vi "getImageinfo.vi"(8 "error in (no error)":errorcluster, 11 "params":refnum<class "JSON Value.lvclass">) -> (0 "error out":errorcluster, 3 "data":refnum<class "JSON Value.lvclass">)   [LabVIEW 2017]
uses:
  <vilib>/NI/JSON Support for LabVIEW/JSON Value/JSON Value.lvclass
  ax5.lvclass
  <vilib>/NI/JSON Support for LabVIEW/JSON Value/Object/Get Value/Get Value (String).vi
  <vilib>/NI/JSON Support for LabVIEW/JSON Value/Object/Get Value/Get Value (Numeric).vi
  <vilib>/NI/JSON Support for LabVIEW/JSON Value/New JSON Value/New JSON (Numeric).vi
  <vilib>/NI/JSON Support for LabVIEW/JSON Value/New JSON Value/New JSON (Numeric[]).vi
  <vilib>/NI/JSON Support for LabVIEW/JSON Value/New JSON Value/New JSON ({Value[]}).vi
  <vilib>/NI/NI JSONRPC Server Framework/Classes/Server/JSONRPC Server.lvclass
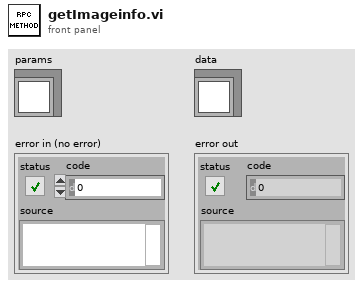
[diagram p1: front panel]
types:
  T1 = typedef "Image Type" = u32
  T2 = cluster{"histogram":u32[], "Minimal Value":sgl, "Maximal Value":sgl, "Starting Value":sgl, "Interval Width":sgl, "Mean Value":sgl, "Standard  Variation":sgl, "Area (pixels)":i32}
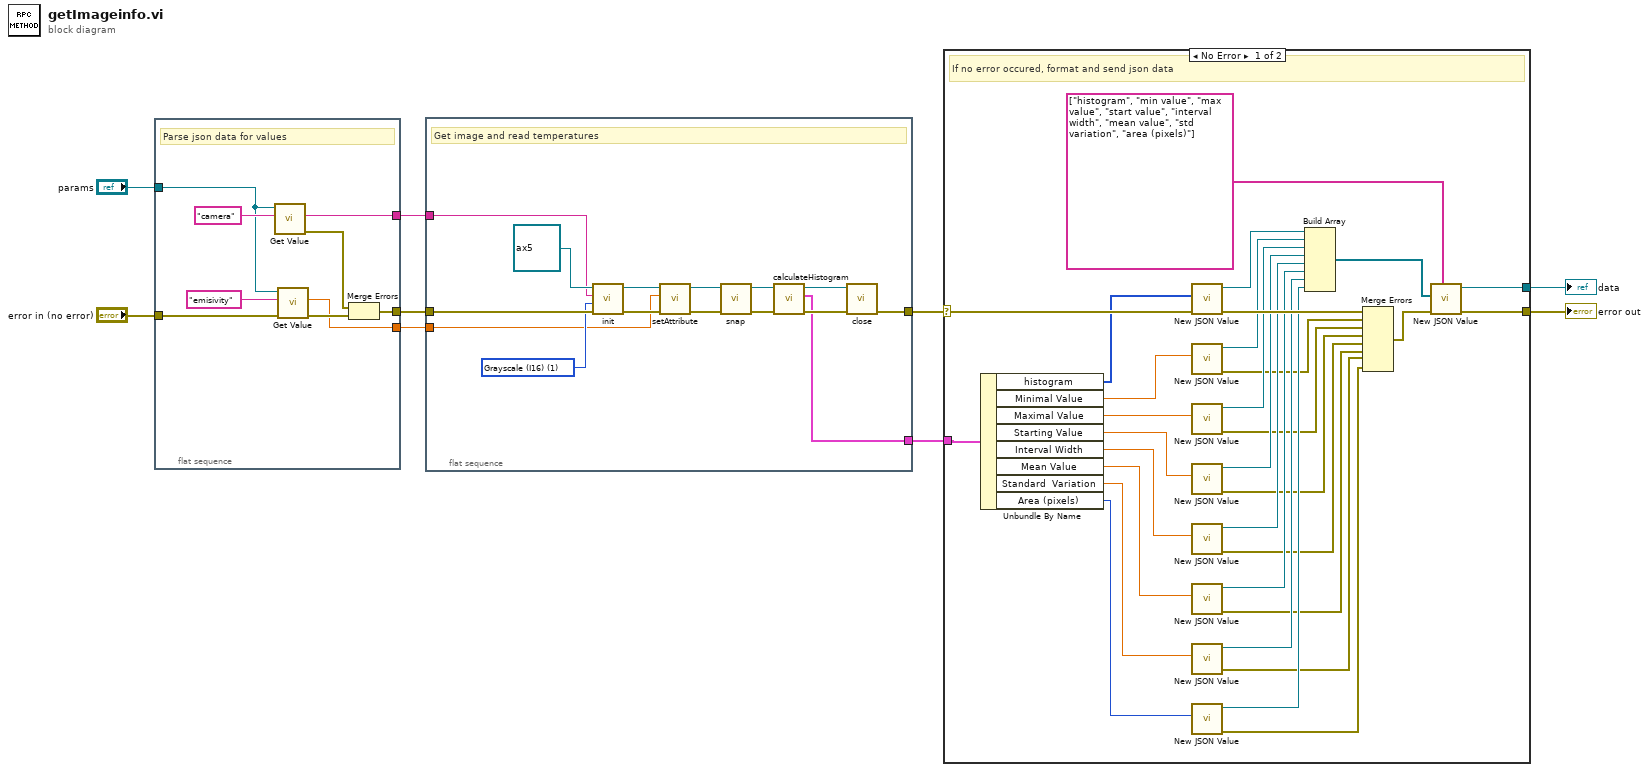
[diagram p0: block diagram]
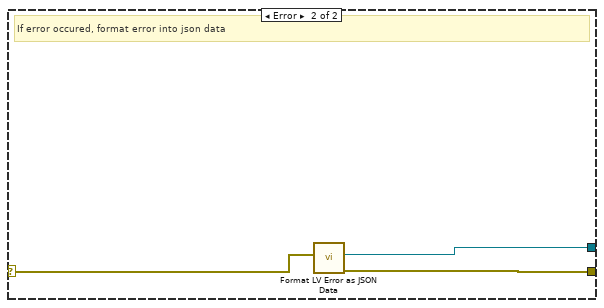
[diagram p2: hidden frame]
diagram:
  n1 = flat-sequence {
    tunnel: "params" -> [w16]
    tunnel: "error in (no error)" -> [w15]
    tunnel: [w12] -> w7
    tunnel: [w11] -> w6
    tunnel: [w10] -> w5
    frame #0 {
      # "Parse json data for values"
      n2 = call-poly <vilib>:"Get Value.vi"("key"="camera", "JSON Value in"=w16) -> ("error out"=w13:errorcluster, "value"=w11:string)  [unwired: 8 in]
      n3 = call-poly <vilib>:"Get Value.vi"("error in (no error)"=w15, "key"="emisivity", "JSON Value in"=w16) -> ("error out"=w14:errorcluster, "value"=w10:dbl)  [unwired: 7 in]
      n4 = Merge Errors(w13, w14) -> (w12:errorcluster)
    }
  }
  n5 = flat-sequence {
    tunnel: w7 -> [w33]
    tunnel: w6 -> [w31]
    tunnel: w5 -> [w27]
    tunnel: [w24] -> w4
    tunnel: [w19] -> w1
    frame #0 {
      w30 = T1 1 items=["Grayscale (U8)", "Grayscale (I16)", "Grayscale (SGL)", "Complex (CSG)", "RGB (U32)", "HSL (U32)", "RGB (U64)", "Grayscale (U16)"] ("Image Type")
      # "Get image and read temperatures"
      n6 = call-dynamic "init.vi"("error in (no error)"=w33, "Image Type"=w30, "Camera Name"=w31, "ax5 in"=refnum<class "ax5.lvclass"> refnum ("ax5.lvclass")) -> ("error out"=w29:errorcluster, "ax5 out"=w28:refnum<class "ax5.lvclass">)  [unwired: 6 in]
      n7 = call-dynamic "setAttribute.vi"("error in (no error)"=w29, "Emissivity"=w27, "ax5.lvclass"=w28) -> ("error out"=w25:errorcluster, "ax5.lvclass"=w26:refnum<class "ax5.lvclass">)  [unwired: 7 in]
      n8 = call-dynamic "snap.vi"("error in (no error)"=w25, "camera in"=w26) -> ("error out"=w23:errorcluster, "camera out"=w22:refnum<class "ax5.lvclass">)  [unwired: 7 in, 1 out]
      n9 = call-dynamic "calculateHistogram.vi"("error in (no error)"=w23, "ax5 in"=w22) -> ("error out"=w21:errorcluster, "tempHistogram"=w19:T2, "ax5 out"=w20:refnum<class "ax5.lvclass">)  [unwired: 7 in]
      n10 = call-dynamic "close.vi"("error in (no error)"=w21, "camera in"=w20) -> ("error out"=w24:errorcluster)  [unwired: 8 in, 1 out]
    }
  }
  n11 = case shown="No Error" w4 {
    selector: w4 -> [w61 w67]
    tunnel: [w63 w65] -> w3
    tunnel: [w60 w66] -> w2
    tunnel: w1 -> [w57 _]
    frame No Error {
      # "If no error occured, format and send json data"
      n12 = Unbundle By Name(w57) -> ("histogram"=w51:u32[], "Minimal Value"=w50:sgl, "Maximal Value"=w49:sgl, "Starting Value"=w52:sgl, "Interval Width"=w53:sgl, "Mean Value"=w54:sgl, "Standard  Variation"=w55:sgl, "Area (pixels)"=w56:i32)
      n13 = call-poly <vilib>:"New JSON Value.vi"("error in (no error)"=w61, "Numeric Array"=w51) -> ("error out"=w64:errorcluster, "JSON Value out"=w41:refnum<class "JSON Value.lvclass">)  [unwired: 8 in]
      n14 = call-poly <vilib>:"New JSON Value.vi"("value"=w50) -> ("error out"=w40:errorcluster, "JSON Value out"=w42:refnum<class "JSON Value.lvclass">)  [unwired: 9 in]
      n15 = call-poly <vilib>:"New JSON Value.vi"("value"=w49) -> ("error out"=w39:errorcluster, "JSON Value out"=w43:refnum<class "JSON Value.lvclass">)  [unwired: 9 in]
      n16 = call-poly <vilib>:"New JSON Value.vi"("value"=w52) -> ("error out"=w38:errorcluster, "JSON Value out"=w44:refnum<class "JSON Value.lvclass">)  [unwired: 9 in]
      n17 = call-poly <vilib>:"New JSON Value.vi"("value"=w53) -> ("error out"=w37:errorcluster, "JSON Value out"=w45:refnum<class "JSON Value.lvclass">)  [unwired: 9 in]
      n18 = call-poly <vilib>:"New JSON Value.vi"("value"=w54) -> ("error out"=w36:errorcluster, "JSON Value out"=w46:refnum<class "JSON Value.lvclass">)  [unwired: 9 in]
      n19 = call-poly <vilib>:"New JSON Value.vi"("value"=w55) -> ("error out"=w35:errorcluster, "JSON Value out"=w47:refnum<class "JSON Value.lvclass">)  [unwired: 9 in]
      n20 = call-poly <vilib>:"New JSON Value.vi"("value"=w56) -> ("error out"=w34:errorcluster, "JSON Value out"=w48:refnum<class "JSON Value.lvclass">)  [unwired: 9 in]
      n21 = Build Array(w41, w42, w43, w44, w45, w46, w47, w48) -> (w59:refnum<class "JSON Value.lvclass">[])
      n22 = Merge Errors(w64, w40, w39, w38, w37, w36, w35, w34) -> (w62:errorcluster)
      n23 = call-poly <vilib>:"New JSON Value.vi"("keys"=string[] ["histogram", "min value", "max value", "start value", "interval width", "mean value", "std variation", "area (pixels)"], "error in (no error)"=w62, "values"=w59) -> ("error out"=w63:errorcluster, "JSON Value out"=w60:refnum<class "JSON Value.lvclass">)  [unwired: 7 in]
    }
    frame Error {
      # "If error occured, format error into json data"
      n24 = call <vilib>:"Format LV Error as JSON Data.vi"("error in"=w67) -> ("error out"=w65:errorcluster, "Error Value out"=w66:refnum<class "JSON Value.lvclass">)  [unwired: 9 in]
    }
  }
  "data" <- w2
  "error out" <- w3
